vi "Raise Done Event.vi"(0 "Raiser Name":string, 5 "Raiser Id":string, 7 "Send Done":bool=TRUE, 9 "Priority":T1, 11 "error in (no error)":errorcluster) -> (15 "error out":errorcluster)   [LabVIEW 2023, in "HAF.lvlib"]
doc: "Helper member to send a Done Event if the passed boolean is True. It is sent at the requested priority."
uses:
  HAF.lvlib
  Event Data.ctl
  Done Event.ctl
  <vilib>/event_ctls.llb/usereventprio.ctl
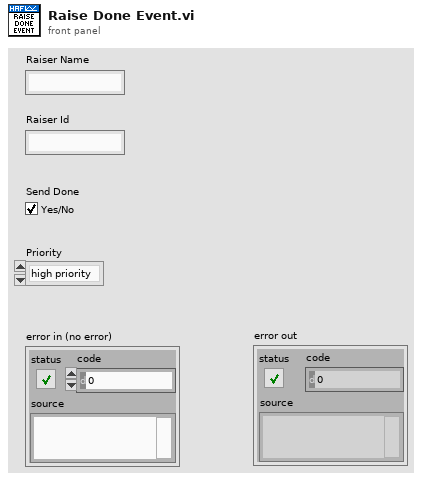
[diagram p1: front panel]
types:
  T1 = typedef "usereventprio.ctl" = enum32{"high priority", "normal priority"}
  T2 = typedef "HAF.lvlib/Event Data.ctl" = cluster{"Raiser Name":string, "Raiser Id":string}
  T3 = typedef "HAF.lvlib/Done Event.ctl" = refnum<user-event>
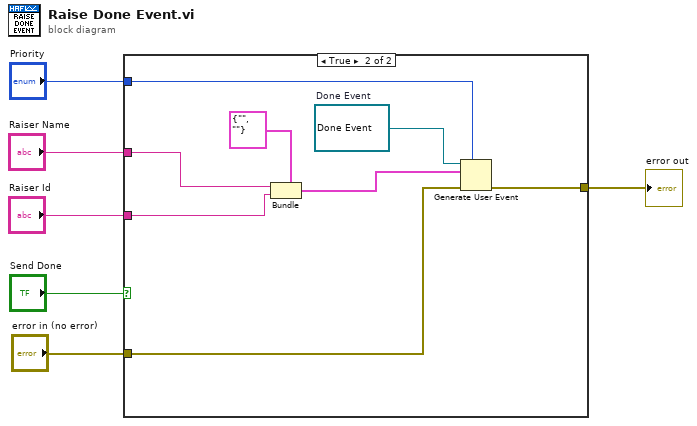
[diagram p0: block diagram]
diagram:
  n1 = case shown="True" "Send Done" {
    tunnel: "error in (no error)" -> [_ w8]
    tunnel: "Priority" -> [_ w13]
    tunnel: "Raiser Name" -> [_ w11]
    tunnel: "Raiser Id" -> [_ w10]
    tunnel: [_ w7] -> w1
    frame False {
    }
    frame True {
      w14 = T3 refnum  # Done Event
      n2 = Bundle(cluster=T2 {"Raiser Name"="", "Raiser Id"=""} ("Event Data Structure"), "Raiser Name"=w11, "Raiser Id"=w10) -> (w9:T2)
      n3 = Generate User Event(priority (normal)=w13, user event=w14, event data cluster=w9, error in=w8) -> (error out=w7:errorcluster)  [unwired: 1 out]
    }
  }
  "error out" <- w1
